vi "moveFrontPanel.vi"(8 "error in (no error)":errorcluster, 11 "VI in":refnum<vi>) -> (0 "error out":errorcluster, 3 "VI out":refnum<vi>)   [LabVIEW 2017, in "QControl_Graph.lvclass"]
uses:
  QControl_Graph.lvclass
  <vilib>/Utility/inputDevices.llb/mouseAcquire.vi
  <vilib>/Utility/inputDevices.llb/closeMouse.vi
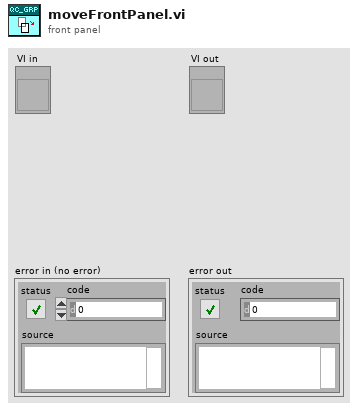
[diagram p1: front panel]
types:
  T1 = cluster{"Horizontal":i32, "Vertical":i32, "Scrolling":i32}
  T2 = typedef "LVRectTypeDef.ctl" = cluster{"Left":i16, "Top":i16, "Right":i16, "Bottom":i16}
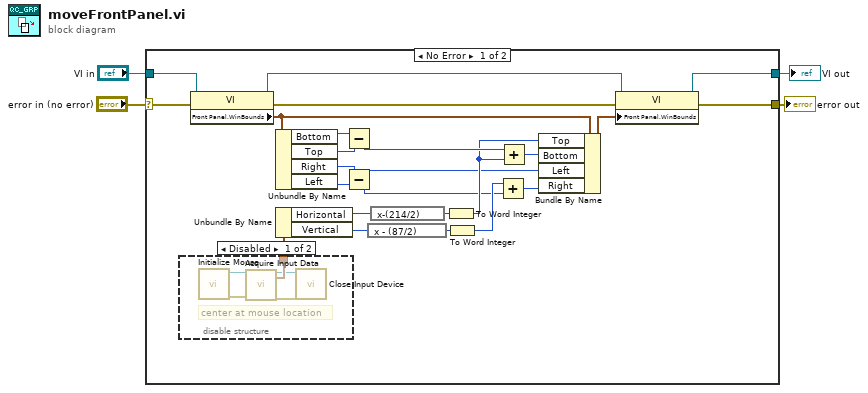
[diagram p0: block diagram]
diagram:
  n1 = case shown="No Error" "error in (no error)" {
    selector: "error in (no error)" -> [w22 w34]
    tunnel: "VI in" -> [w27 w33]
    tunnel: [w26 w34] -> w3
    tunnel: [w24 w33] -> w2
    frame No Error {
      n2 = disable-structure shown="Disabled" {
        disable-tunnel: [w32 _] -> w21
        frame Disabled {
          # "center at mouse location"
          n3 = call <vilib>:"Initialize Mouse.vi"() -> ("error out"=w29:errorcluster, "device ID"=w31:refnum<k1>)  [unwired: 10 in]
          n4 = call-poly <vilib>:"Acquire Input Data.vi"("device ID"=w31, "error in (no error)"=w29) -> ("device ID"=w30:refnum<k1>, "axis info"=w32:T1, "error out"=w28:errorcluster)  [unwired: 14 in, 1 out]
          n5 = call-poly <vilib>:"Close Input Device.vi"("error in (no error)"=w28, "device ID"=w30) -> ()  [unwired: 8 in, 1 out]
        }
        frame Enabled {
        }
      }
      n6 = property class="VI"(reference=w27, error in=w22) -> (reference out=w25:refnum<vi>, error out=w23:errorcluster, "Front Panel.WinBounds"=w15:T2)
      n7 = Unbundle By Name(w15) -> ("Bottom"=w13:i16, "Top"=w14:i16, "Right"=w12:i16, "Left"=w11:i16)
      n8 = Unbundle By Name(w21) -> ("Horizontal"=w18:i32, "Vertical"=w19:i32)
      n9 = Subtract(x=w13, y=w14) -> (x-y=w10:i16)
      n10 = Subtract(x=w12, y=w11) -> (x-y=w5:i16)
      n11 = expression code="x - (87/2)"(w19) -> (w17:i32)
      n12 = expression code="x-(214/2)"(w18) -> (w20:i32)
      n13 = To Word Integer(number=w20) -> (16bit integer=w9:i16)
      n14 = To Word Integer(number=w17) -> (16bit integer=w6:i16)
      n15 = Add(x=w6, y=w5) -> (x+y=w7:i16)
      n16 = Add(x=w10, y=w9) -> (x+y=w8:i16)
      n17 = Bundle By Name(cluster=w15, "Top"=w9, "Bottom"=w8, "Left"=w5, "Right"=w7) -> (w16:T2)
      n18 = property class="VI"(reference=w25, error in=w23, "Front Panel.WinBounds"=w16) -> (reference out=w24:refnum<vi>, error out=w26:errorcluster)
    }
    frame Error {
    }
  }
  "error out" <- w3
  "VI out" <- w2
